vi "Sortowanie po promieniu.vi"(2 "error in":errorcluster, 3 "unsorted array":dbl[][](array[numeric])) -> (0 "error out":errorcluster, 1 "Array 2":dbl[][][](array[numeric]))   [LabVIEW 2016]
doc: "To vi sortuje tablice 1d pkt w tablice 2d pkt względem promienia , gdzie każdy wiersz to pkt z tym samym promieniem"
uses:
  <vilib>/express/express arith-compare/Formula/XNode/ExpressFormulaBlockNode.xnode
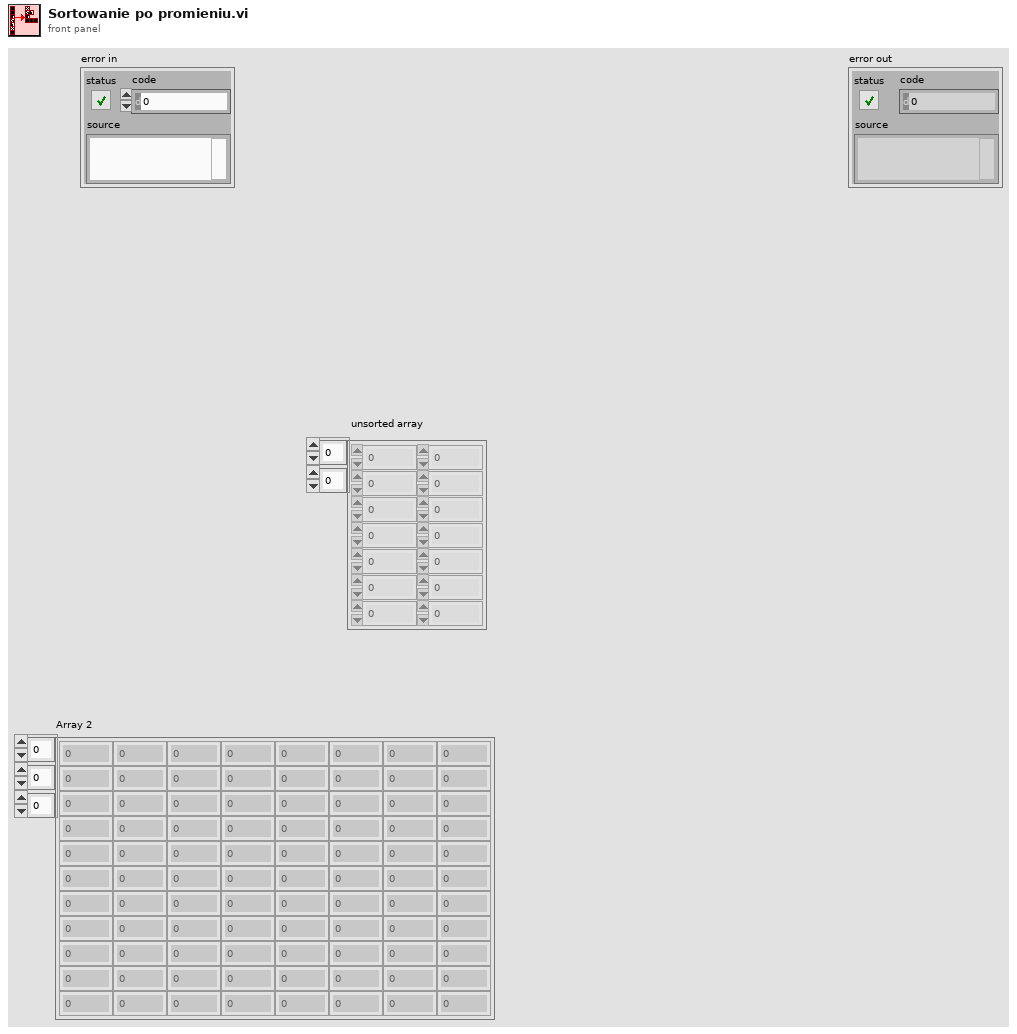
[diagram p1: front panel]
types:
  T1 = cluster{"Result":dbl, "Numeric":dbl, "Numeric":dbl}
  T2 = cluster{"Result":dbl, "Numeric":dbl, "Numeric":dbl}[]
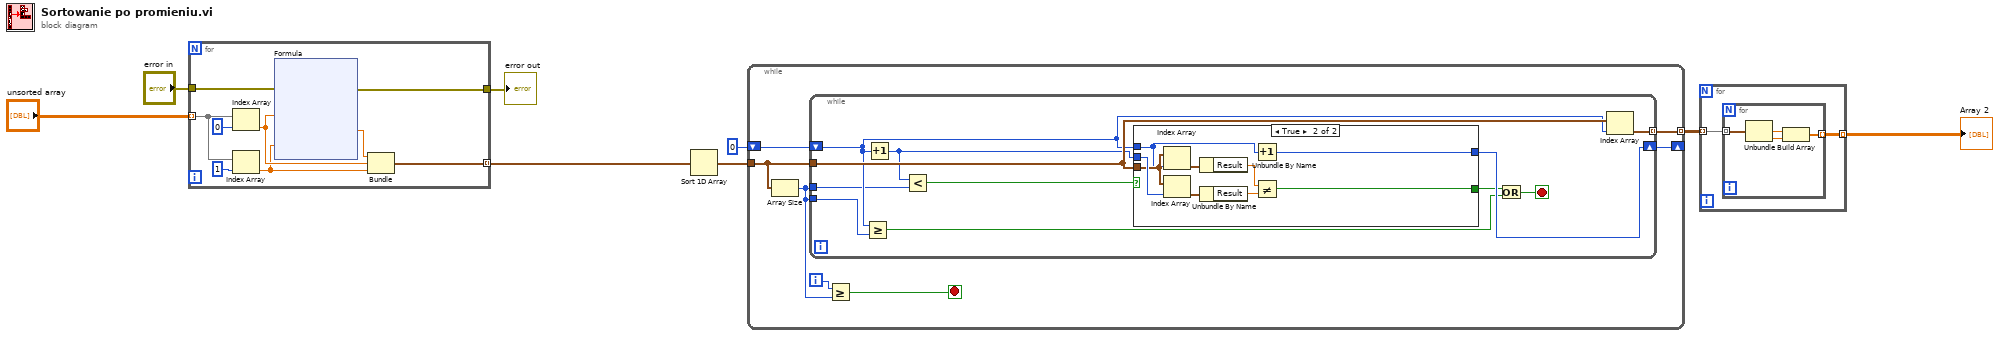
[diagram p0: block diagram]
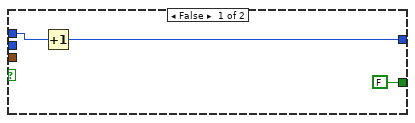
[diagram p2: hidden frame]
diagram:
  n1 = for {
    tunnel: "unsorted array" -> [w14] mode=indexing
    tunnel: [w15] -> w5 mode=indexing
    tunnel: "error in" -> [w13]
    tunnel: [w12] -> w6
    n2 = Index Array(array=w14, index=0) -> (element=w11:dbl)
    n3 = Index Array(array=w14, index=1) -> (element=w10:dbl)
    n4 = xnode "Formula"("x"=w11, "y"=w10, "error in (no error)"=w13) -> ("Result"=w9:dbl, "error out"=w12:errorcluster)
    n5 = Bundle("Result"=w9, "Numeric"=w11, "Numeric"=w10) -> (w15:T1)  [unwired: 1 in]
  }
  "error out" <- w6
  n6 = Sort 1D Array(array=w5) -> (sorted array=w4:T2)
  n7 = while {
    tunnel: w4 -> [w32]
    shift-right: [w30] -> _
    shift-left: 0 ("index") -> [w31]
    tunnel: [w29] -> w2 mode=indexing
    i -> [w34]
    stop <- w33 stop-if-true
    n8 = Array Size(array=w32) -> (size(s)=w28:i32)
    n9 = while {
      tunnel: w32 -> [w43]
      shift-right: [w41] -> w30
      shift-left: w31 -> [w39]
      tunnel: [w45] -> w29 mode=indexing
      tunnel: w28 -> [w40]
      tunnel: w28 -> [w35]
      stop <- w36 stop-if-true
      n10 = Greater Or Equal?(x=w39, y=w40) -> (x >= y?=w38:bool)
      n11 = Increment(x=w39) -> (x+1=w42:i32)
      n12 = Less?(x=w42, y=w35) -> (x < y?=w44:bool)
      n13 = case shown="True" w44 {
        tunnel: w43 -> [_ w56]
        tunnel: w39 -> [w46 w49]
        tunnel: w42 -> [_ w57]
        tunnel: [w47 w55] -> w41
        tunnel: [FALSE w50] -> w37
        frame False {
          n14 = Increment(x=w46) -> (x+1=w47:i32)
        }
        frame True {
          n15 = Index Array(array=w56, index=w49) -> (element=w54:T1)
          n16 = Index Array(array=w56, index=w57) -> (element=w53:T1)
          n17 = Unbundle By Name(w54) -> ("Result"=w52:dbl)
          n18 = Unbundle By Name(w53) -> ("Result"=w51:dbl)
          n19 = Increment(x=w49) -> (x+1=w55:i32)
          n20 = Not Equal?(x=w52, y=w51) -> (x != y?=w50:bool)
        }
      }
      n21 = Or(x=w37, y=w38) -> (x .or. y?=w36:bool)
      n22 = Index Array(array=w43, index=w39) -> (element=w45:T1)
    }
    n23 = Greater Or Equal?(x=w34, y=w28) -> (x >= y?=w33:bool)
  }
  n24 = for {
    tunnel: w2 -> [w59] mode=indexing
    tunnel: [w58] -> w1 mode=indexing
    n25 = for {
      tunnel: w59 -> [w63] mode=indexing
      tunnel: [w60] -> w58 mode=indexing
      n26 = Unbundle(w63) -> ("Numeric"=w62:dbl, "Numeric"=w61:dbl)  [unwired: 1 out]
      n27 = Build Array(w62, w61) -> (w60:dbl[])
    }
  }
  "Array 2" <- w1
